vi "TimeInterpVariant_Interpolate.vi"(6 "Extra Data":variant, 9 "Time Fraction":dbl, 10 "Input 2":variant, 11 "Input 1":variant) -> (3 "Interp Output":variant)   [LabVIEW 2019, in "Trajectory_Library.lvlib"]
uses:
  Trajectory_Library.lvlib
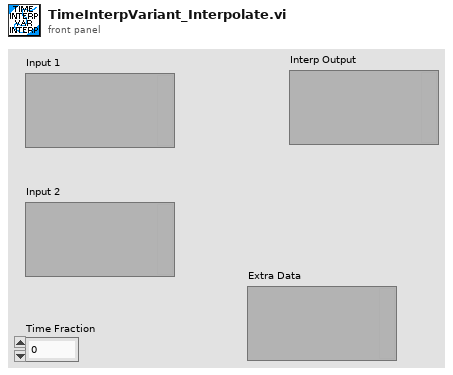
[diagram p1: front panel]
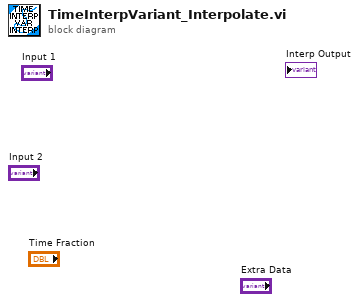
[diagram p0: block diagram]
diagram:
